vi "cvi_photons_in_bins.vi"(4 "offset_lag":dbl, 5 "stop_time_ps":dbl, 6 "coarseness":dbl, 7 "start_time_ps":dbl, 8 "error in (no error)":errorcluster, 10 "ch2":dbl[](array[numeric]), 11 "ch1":dbl[](array[numeric])) -> (0 "error out":errorcluster, 2 "lags":dbl[](array[numeric]), 3 "acf":dbl[](array[numeric]))   [LabVIEW 2015]
uses:
  cvibuild.corr_funcs/Release/corr_funcs.dll
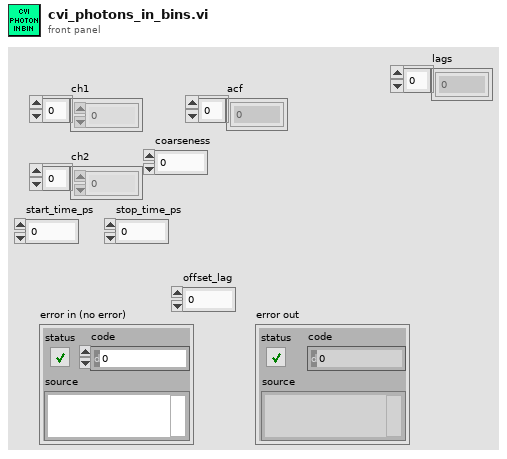
[diagram p1: front panel]
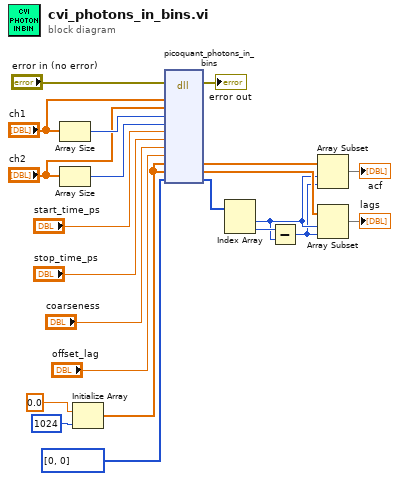
[diagram p0: block diagram]
diagram:
  n1 = Array Size(array="ch1") -> (size(s)=w20:i32)
  n2 = Array Size(array="ch2") -> (size(s)=w18:i32)
  n3 = Initialize Array(0.0 ("element"), 1024 ("dimension size")) -> (w10:dbl[])
  n4 = dll-call lib="C:/Users/bspoka/Downloads/lvoop_dll-master/cvi_project/cvibuild.corr_funcs/Release/corr_funcs.dll" fn="picoquant_photons_in_bins"(error in="error in (no error)", "ch1"="ch1", "ch2"="ch2", "num_ch1"=w20, "num_ch2"=w18, "start_time_ps"="start_time_ps", "stop_time_ps"="stop_time_ps", "coarseness"="coarseness", "offset_lag_ps"="offset_lag", "acf"=w10, "lags"=w10, "acf_length"=i32[] [0, 0]) -> (error out=→"error out":errorcluster, "acf"=w8:dbl[], "lags"=w4:dbl[], "acf_length"=w7:i32[])  [unwired: 11 in, 1 out]
  n5 = Index Array(array=w7) -> (element #1=w2:i32, element #2=w6:i32)  [unwired: 2 in]
  n6 = Subtract(x=w6, y=w2) -> (x-y=w1:i32)
  n7 = Array Subset(array=w8, index=w2, length=w1) -> (→"acf":dbl[])
  n8 = Array Subset(array=w4, index=w2, length=w1) -> (→"lags":dbl[])
